vi "000_DataEmulator.vi"(11 "Queue Ref In":T1={"UI"=refnum, "Message"=refnum, "Data"=refnum, "Caller"=refnum, "Name"="000 Common", "Data Path"=path "", "Class Path"=path "", "SubPanel"=refnum, "Project Name"="", "MNT"="", "Title"="", "Data Source"=refnum, "Queue List"={}, "VI"=refnum, "UE"=refnum}) -> ()   [LabVIEW 2020]
doc: "000_DataEmulator.vi"
uses:
  Alin/QMH/000 Module Data Type.ctl
  Alin/QMH/Queue Message.ctl
  9999 SubVI/Global/Data Global/SDQ Data Type.ctl
  <vilib>/Utility/miscctls.llb/LVRowAndColumnUnsignedTypeDef.ctl
panel:
  in  "Delete":bool
  in  "Export":bool
  in  "Data Load":bool
  in  "Source Edit":bool
  out "Num":i32
  in  "Input":string
  in  "Panel Show":bool
  in  "Source List":i32[](listbox)
  in  "Delay(ms)":u32(slide)=250 min=5 max=2000 step=1 scale=5.0..2000.0
  in  "Simulation Start":bool
  in  "Data List":i32(listbox)
  out "Name":string
  out "Active ID":string
  out "Type":enum32{"decimal", "bool"}(tab)
  out "Unit":string
  in  "Type":enum16{"Sin"}(ring)
  in  "Single Simulation Start":bool
  in  "Value":sgl(slide)=250.0 min=0 max=1 scale=0.0..1.0 scale format="%#.6f"
  in  "Bool":bool
  out "Data":T2
  out "Count":u32
  out "Elapsed time(ms)":u32
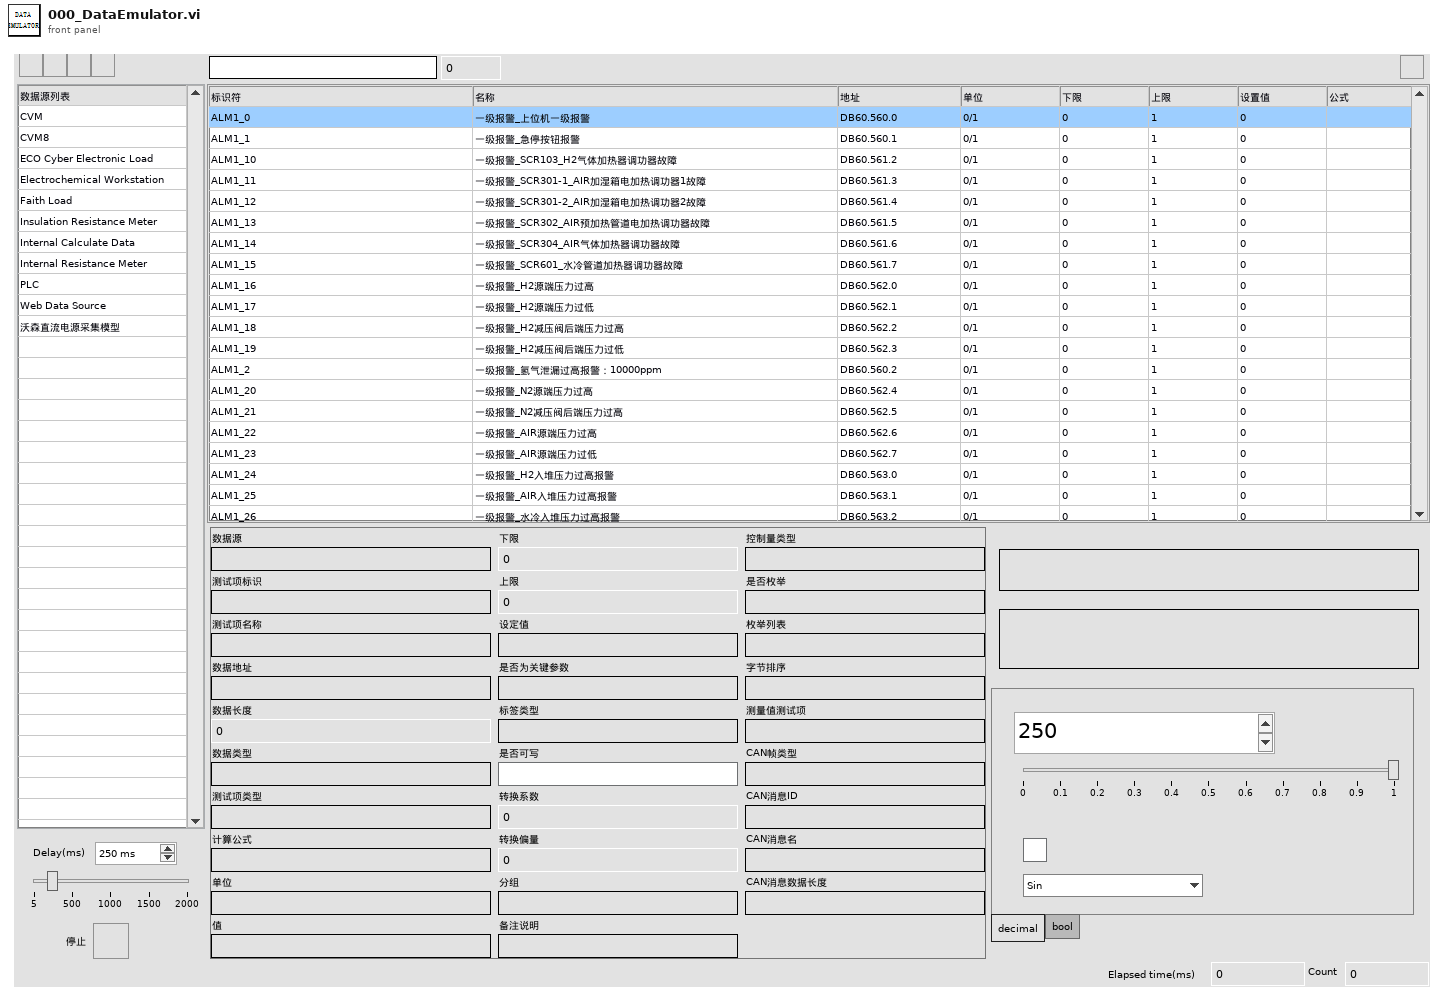
[diagram p1: front panel]
types:
  T1 = typedef "000 Module Data Type.ctl" = cluster{"UI":refnum<queue>, "Message":refnum<queue>, "Data":refnum<queue>, "Caller":refnum<queue>, "Name":string, "Data Path":path, "Class Path":path, "SubPanel":refnum<vi>, "Project Name":string, "MNT":string, "Title":string, "Data Source":refnum<queue>, "Queue List":map{string, refnum<queue>}, "VI":refnum<vi>, "UE":refnum<user-event>}
  T2 = typedef "SDQ Data Type.ctl" = cluster{"CAN Length":string, "CAN Name":string, "CAN ID":string, "CAN Type":string, "Test Item":string, "Byte Order":string, "Instruction":string, "Control Type":string, "Group":string, "Offset":dbl, "Coefficient":dbl, "Write Enable":bool, "Lable Type":string, "Key?":string, "Set Value":string, "Upper":dbl, "Lower":dbl, "Unit":string, "Formula":string, "Test Item Type":string, "Length":i32, "Address":string, "Name":string, "Identifier":string, "Data Type":string, "Enumerate?":string, "Enumerate List":string, "Data":string, "Source":string}
  T3 = typedef "LVRowAndColumnUnsignedTypeDef.ctl" = cluster{"Row":u32, "Column":u32}
  T4 = cluster{"Queue":T1, "Delay":cluster{"Count Time(ms)":u32, "Delay Time(ms)":u32, "Next":string}, "Data":map{string, T2}, "Start":bool, "Type":map{string, string}, "Source List":refnum<vi>, "TData":map{string, T2}, "Title":string[], "Source":map{string, string[]}, "Data List":refnum<vi>, "Value":refnum<vi>, "AID":string}
  T5 = cluster{"Name":string, "Type":map{string, string}}
  T6 = typedef "eventvkey.ctl" = enum16{"ASCII", "Enter", "Return", "Shift", "Ctrl", "Alt", "Cmd", "Opt", "Caps", "NumLock", "Clear", "Break", "Up", "Down", "Left", "Right", "Insert", "Delete", "Home", "End", "PageUp", "PageDown", "Escape", "Help", "Pause", "ScrollLock", "F1", "F2", "F3", "F4", "F5", "F6", "F7", "F8", "F9", "F10", "F11", "F12", "F13", "F14", "F15", "F16", "F17", "F18", "F19", "F20", "F21", "F22", "F23", "F24", "Play", "VolumeUp", "VolumeDown", "Mute", "Two Byte Char"}
  T7 = cluster{"Shift":bool, "Ctrl":bool, "Alt":bool, "Cmd":bool, "Opt":bool}
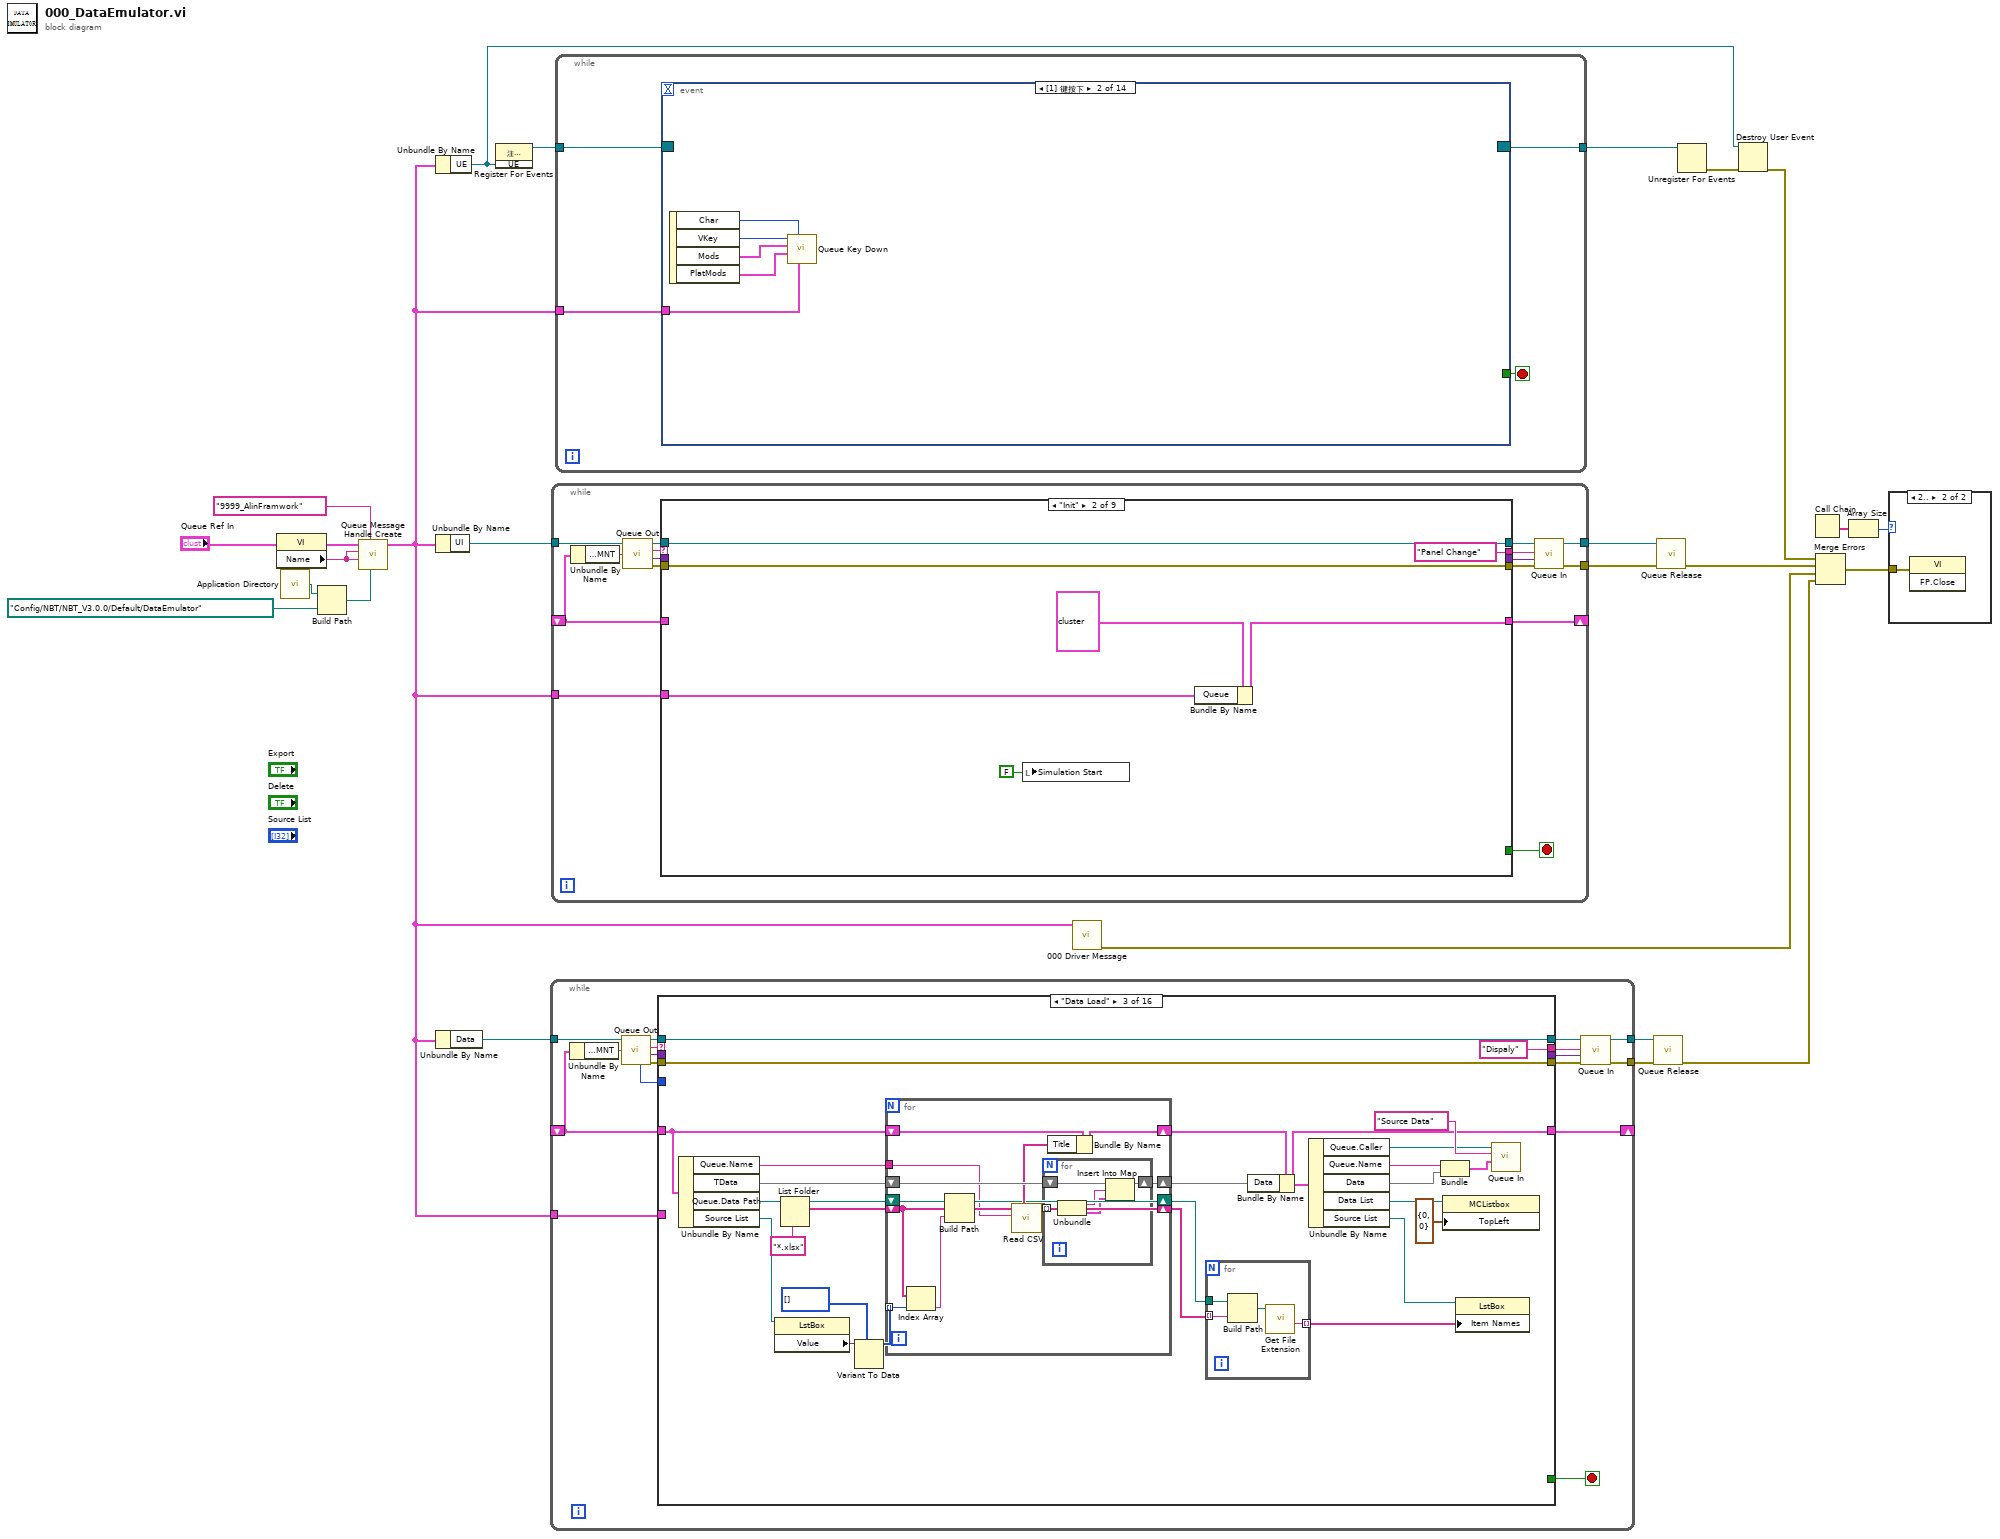
[diagram p0: block diagram]
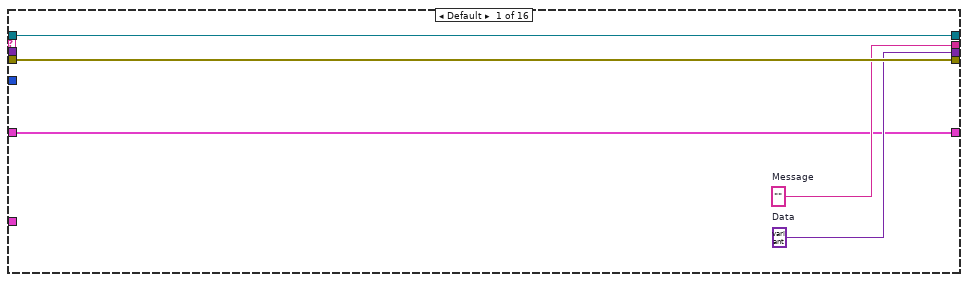
[diagram p2: hidden frame]
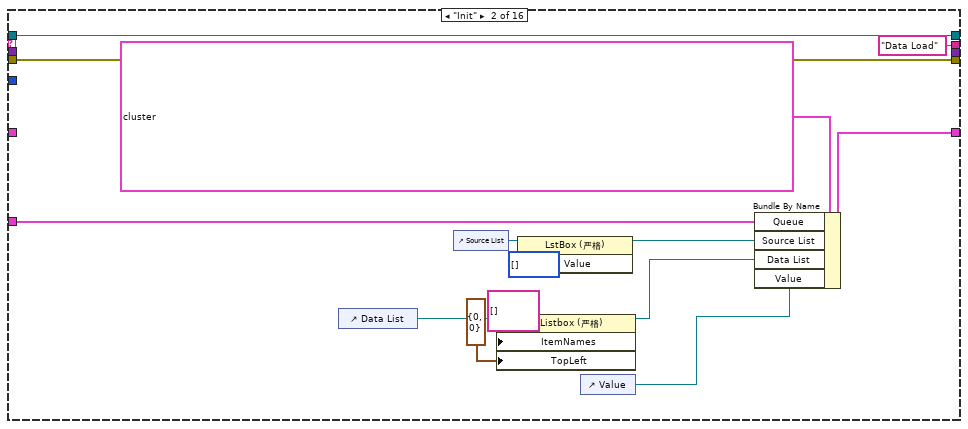
[diagram p3: hidden frame]
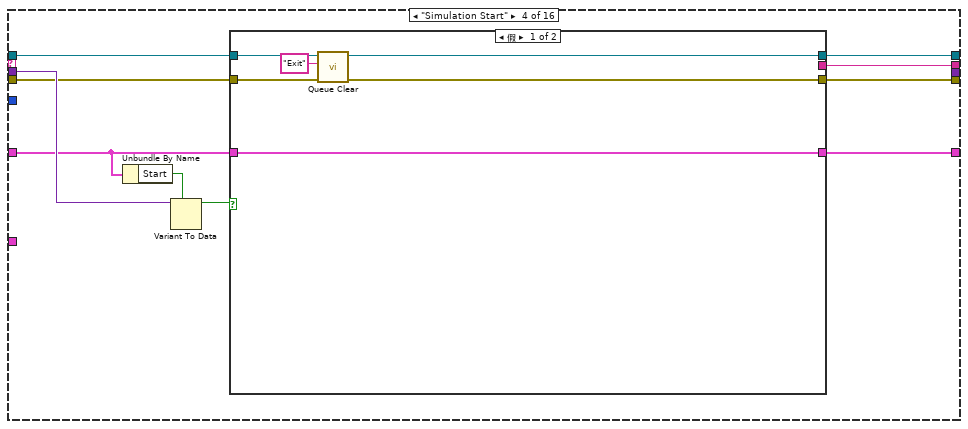
[diagram p4: hidden frame]
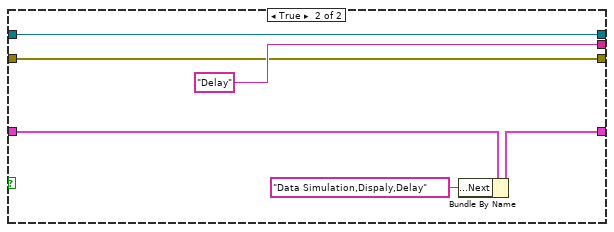
[diagram p5: hidden frame]
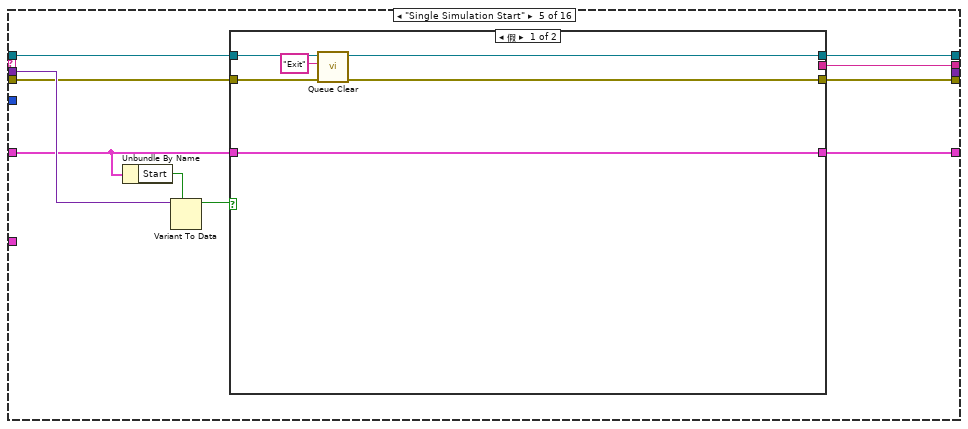
[diagram p6: hidden frame]
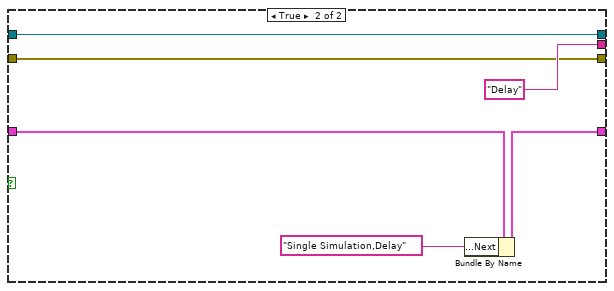
[diagram p7: hidden frame]
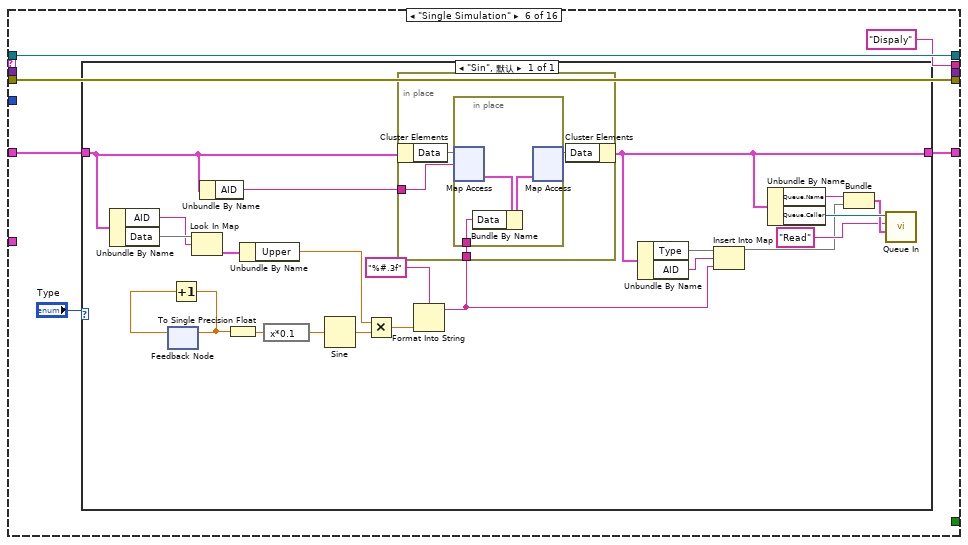
[diagram p8: hidden frame]
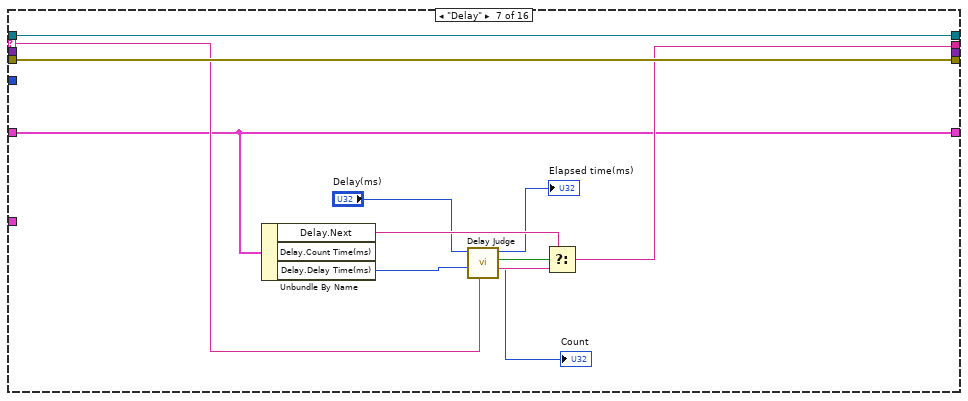
[diagram p9: hidden frame]
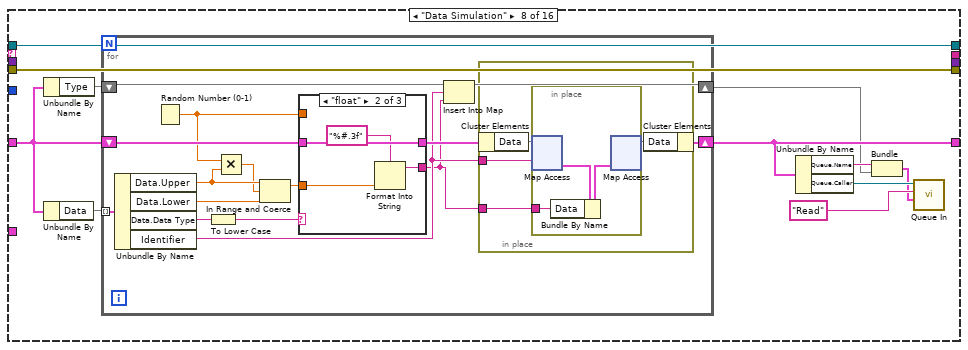
[diagram p10: hidden frame]
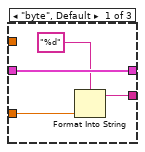
[diagram p11: hidden frame]
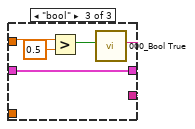
[diagram p12: hidden frame]
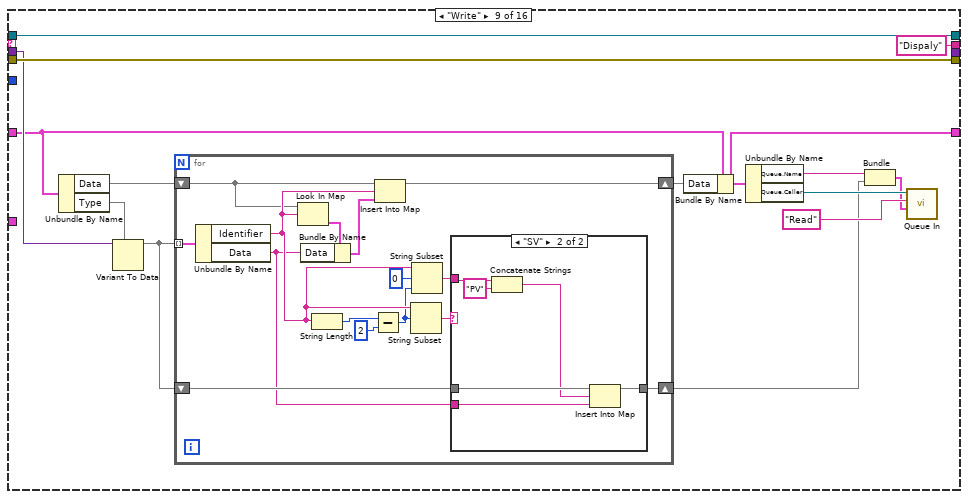
[diagram p13: hidden frame]
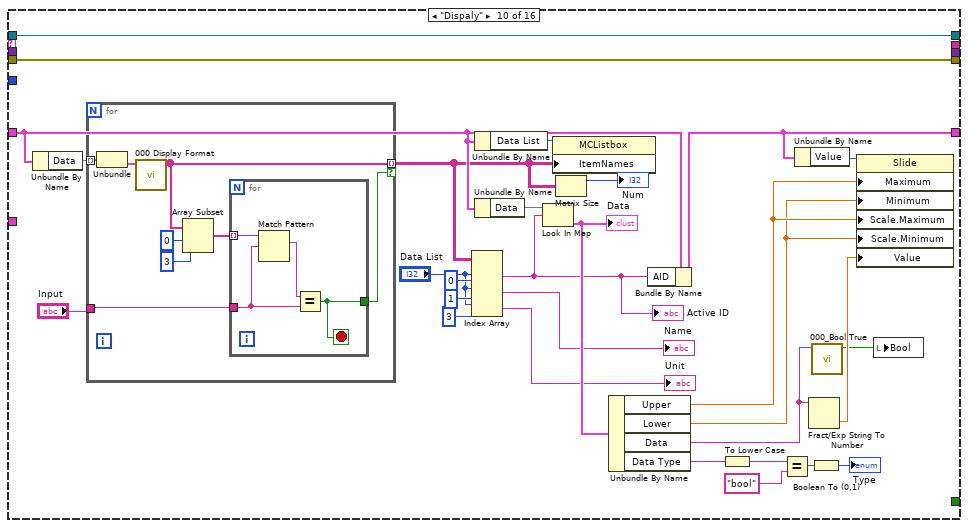
[diagram p15: hidden frame]
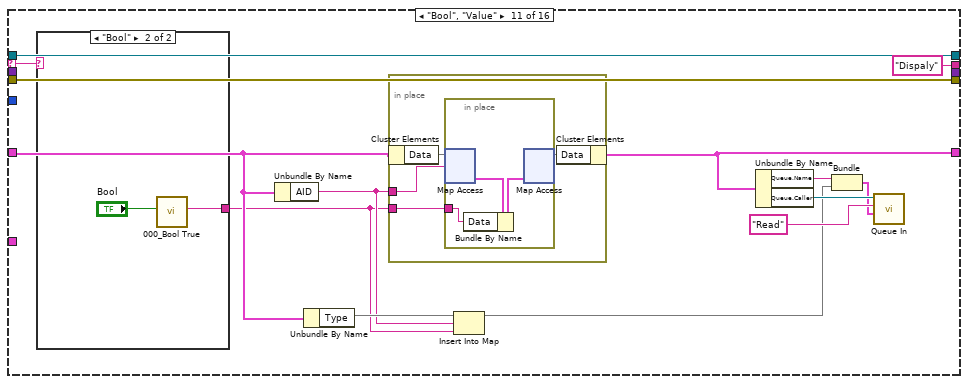
[diagram p16: hidden frame]
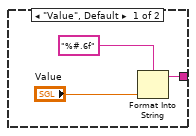
[diagram p17: hidden frame]
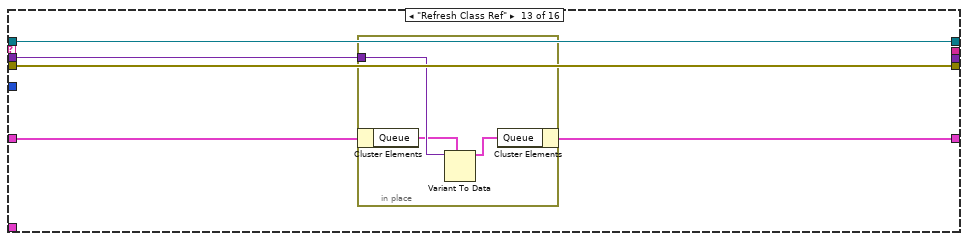
[diagram p19: hidden frame]
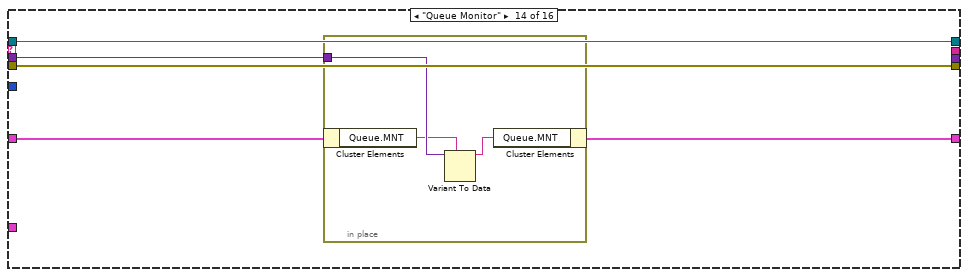
[diagram p20: hidden frame]
diagram:
  n1 = property class="VI"() -> ("Name"=w5:string)  [unwired: 2 in, 2 out]
  n2 = call <vilib>:"Application Directory.vi"() -> ("Application Directory"=w3:path)
  n3 = Build Path(base path=w3, name or relative path=path "Config/NBT/NBT_V3.0.0/Default/DataEmulator" ("名称或相对路径")) -> (appended path=w1:path)
  n4 = call "Queue Message Handle Create.vi"("Data Path"=w1, "Project Name"="9999_AlinFramwork", "Name"=w5, "Title"=w5, "Queue Ref In"="Queue Ref In") -> ("Queue Ref Out"=w6:T1)  [unwired: 5 in, 1 out]
  n5 = Unbundle By Name(w6) -> ("UE"=w8:refnum<user-event>)
  n6 = Unbundle By Name(w6) -> ("UI"=w19:refnum<queue>)
  n7 = Unbundle By Name(w6) -> ("Data"=w11:refnum<queue>)
  n8 = register-events(w8) -> (reference out=w24:refnum<event-registration>)  [unwired: 2 in, 1 out]
  n9 = while {
    tunnel: w11 -> [w37]
    tunnel: [w34] -> w13
    tunnel: [w33] -> w12
    shift-right: [w29] -> _
    shift-left: _ -> [w26]
    tunnel: w6 -> [w25]
    stop <- w41 stop-if-true
    n10 = Unbundle By Name(w26) -> ("Queue.MNT"=w27:string)
    n11 = call "Queue Out.vi"("Monitor"=w27, "Queue In"=w37) -> ("error out"=w40:errorcluster, "Data"=w38:variant, "Message"=w39:string, "Queue Out"=w36:refnum<queue>, "Queue NUmber"=w28:i32)  [unwired: 5 in]
    n12 = case shown="\"Data Load\"" w39 {
      selector: w39 -> [_ _ _ _ _ _ w193 _ _ _ w335 _ _ _ _ _]
      tunnel: w36 -> [w46 w60 w65 w116 w138 w159 w199 w210 w260 w311 w337 w352 w357 w365 w373 w377]
      tunnel: w40 -> [w45 w59 w88 w114 w136 w158 w198 w209 w259 w310 w336 w351 w356 w364 w371 w378]
      tunnel: [w46 w60 w65 w115 w137 w159 w199 w210 w260 w311 w337 w352 w357 w365 w372 w377] -> w35
      tunnel: [w45 w59 w88 w113 w135 w158 w198 w209 w259 w310 w336 w351 w356 w364 w370 w378] -> w32
      tunnel: [w44 "Data Load" ("Next") "Dispaly" ("Next") w117 w139 "Dispaly" ("Next") w194 _ "Dispaly" ("Next") _ "Dispaly" ("Next") _ _ _ "Quit" _] -> w31
      tunnel: [_ _ _ _ _ _ _ _ _ _ _ _ _ _ _ TRUE] -> w41
      tunnel: [w43 _ _ _ _ _ _ _ _ _ _ _ _ _ _ _] -> w30
      tunnel: w38 -> [_ _ _ w119 w141 _ _ _ w258 _ _ _ w353 w361 _ _]
      tunnel: [w42 w56 w73 w110 w132 w155 w192 w205 w248 w296 w330 w350 w354 w362 w369 w375] -> w29
      tunnel: w26 -> [w42 _ w67 w111 w133 w156 w192 w207 w255 w298 w329 w350 w355 w363 w369 w375]
      tunnel: w28 -> [_ _ _ _ _ _ _ _ _ _ _ _ _ _ _ _]
      tunnel: w25 -> [_ w55 _ _ _ _ _ _ _ _ _ _ _ _ _ _]
      frame Default {
        w43 = variant  # Data
        w44 = ""  # Message
      }
      frame "Init" {
        n13 = control-ref of="Data List"() -> (w51:refnum<vi>)
        n14 = control-ref of="Source List"() -> (w54:refnum<vi>)
        n15 = property class="MCListbox (严格)"(reference=w51, "ItemNames"=string[][] [] ("项名"), "TopLeft"=T3 {"Row"=0, "Column"=0} ("左上可见单元格")) -> (reference out=w50:refnum<vi>)  [unwired: 1 in, 1 out]
        n16 = property class="LstBox (严格)"(reference=w54, "Value"=i32[] [] ("值")) -> (reference out=w53:refnum<vi>)  [unwired: 1 in, 1 out]
        n17 = control-ref of="Value"() -> (w47:refnum<vi>)
        n18 = Bundle By Name(cluster=T4 {"Queue"={"UI"=refnum, "Message"=refnum, "Data"=refnum, "Caller"=refnum, "Name"="000 Common", "Data Path"=path "", "Class Path"=path "", "SubPanel"=refnum, "Project Name"="", "MNT"="", "Title"="", "Data Source"=refnum, "Queue List"={}, "VI"=refnum, "UE"=refnum}, "Delay"={"Count Time(ms)"=250, "Delay Time(ms)"=50, "Next"="Data Simulation,Dispaly,Delay"}, "Data"={}, "Start"=FALSE, "Type"={}, "Source List"=refnum, "TData"={}, "Title"=[], "Source"={}, "Data List"=refnum, "Value"=refnum, "AID"=""}, "Queue"=w55, "Source List"=w53, "Data List"=w50, "Value"=w47) -> (w56:T4)
      }
      frame "Data Load" {
        n19 = Unbundle By Name(w67) -> ("Queue.Name"=w72:string, "TData"=w85:map{string, T2}, "Queue.Data Path"=w87:path, "Source List"=w83:refnum<vi>)
        n20 = property class="LstBox"(reference=w83) -> ("Value"=w82:variant)  [unwired: 1 in, 2 out]
        n21 = List Folder(path=w87, pattern="*.xlsx" ("类型")) -> (path out=w86:path, filenames=w79:string[])  [unwired: 2 in, 2 out]
        n22 = Variant To Data(type=i32[] [] ("Source List"), Variant=w82) -> (data=w80:i32[])  [unwired: 1 in, 1 out]
        n23 = for {
          shift-right: [w102] -> w84
          shift-left: w85 -> [w103]
          tunnel: w80 -> [w101] mode=indexing
          tunnel: w72 -> [w93]
          shift-right: [w100] -> w70
          shift-left: w79 -> [w100]
          shift-right: [w95] -> w71
          shift-left: w86 -> [w95]
          shift-right: [w98] -> w66
          shift-left: w67 -> [w99]
          n24 = Index Array(array=w100, index=w101) -> (element=w96:string)
          n25 = Build Path(base path=w95, name or relative path=w96) -> (appended path=w94:path)
          n26 = call "Read CSV.vi"("Source"=w93, "Data Path"=w94) -> ("Identifiers Out"=w104:map{string, T2}, "Title"=w97:string[])  [unwired: 2 in, 6 out]
          n27 = for {
            tunnel: w104 -> [w107] mode=indexing
            shift-right: [w108] -> w102
            shift-left: w103 -> [w109]
            n28 = Unbundle(w107) -> ("Identifier"=w105:string, "Data"=w106:T2)
            n29 = Insert Into Map(map in=w109, key=w105, value=w106) -> (map out=w108:map{string, T2})  [unwired: 2 out]
          }
          n30 = Bundle By Name(cluster=w99, "Title"=w97) -> (w98:T4)
        }
        n31 = for {
          tunnel: w71 -> [w92]
          tunnel: w70 -> [w91] mode=indexing
          tunnel: [w89] -> w69 mode=indexing
          n32 = Build Path(base path=w92, name or relative path=w91) -> (appended path=w90:path)
          n33 = call <vilib>:"Get File Extension.vi"("file"=w90) -> ("filename without extension"=w89:string)  [unwired: 6 in, 4 out]
        }
        n34 = Bundle By Name(cluster=w66, "Data"=w84) -> (w73:T4)
        n35 = Unbundle By Name(w73) -> ("Queue.Caller"=w74:refnum<queue>, "Queue.Name"=w78:string, "Data"=w76:map{string, T2}, "Data List"=w62:refnum<vi>, "Source List"=w63:refnum<vi>)
        n36 = Bundle("Name"=w78, "Data"=w76) -> (w77:cluster{"Name":string, "Data":map{string, T2}})  [unwired: 1 in]
        n37 = property class="MCListbox"(reference=w62, "TopLeft"=T3 {"Row"=0, "Column"=0} ("左上可见单元格")) -> ()  [unwired: 1 in, 2 out]
        n38 = property class="LstBox"(reference=w63, "Item Names"=w69) -> ()  [unwired: 1 in, 2 out]
        n39 = call "Queue In.vi"("Data"=w77, "Message"="Source Data", "Queue In"=w74) -> ()  [unwired: 7 in, 2 out]
      }
      frame "Simulation Start" {
        n40 = Unbundle By Name(w111) -> ("Start"=w112:bool)
        n41 = Variant To Data(type=w112, Variant=w119) -> (data=w118:bool)  [unwired: 1 in, 1 out]
        n42 = case shown="假" w118 {
          tunnel: [_ "Delay" ("Next")] -> w117
          tunnel: w116 -> [w123 w130]
          tunnel: [w122 w130] -> w115
          tunnel: w114 -> [w125 w129]
          tunnel: [w124 w129] -> w113
          tunnel: w111 -> [w120 w128]
          tunnel: [w120 w127] -> w110
          frame False {
            n43 = call "Queue Clear.vi"("error in (no error)"=w125, "Filter"="Exit", "Queue In"=w123) -> ("error out"=w124:errorcluster, "Queue Out"=w122:refnum<queue>)  [unwired: 7 in]
          }
          frame True {
            n44 = Bundle By Name(cluster=w128, "Delay.Next"="Data Simulation,Dispaly,Delay") -> (w127:T4)
          }
        }
      }
      frame "Single Simulation Start" {
        n45 = Unbundle By Name(w133) -> ("Start"=w134:bool)
        n46 = Variant To Data(type=w134, Variant=w141) -> (data=w140:bool)  [unwired: 1 in, 1 out]
        n47 = case shown="假" w140 {
          tunnel: [_ "Delay" ("Next")] -> w139
          tunnel: w138 -> [w145 w152]
          tunnel: [w144 w152] -> w137
          tunnel: w136 -> [w147 w151]
          tunnel: [w146 w151] -> w135
          tunnel: w133 -> [w142 w150]
          tunnel: [w142 w149] -> w132
          frame False {
            n48 = call "Queue Clear.vi"("error in (no error)"=w147, "Filter"="Exit", "Queue In"=w145) -> ("error out"=w146:errorcluster, "Queue Out"=w144:refnum<queue>)  [unwired: 7 in]
          }
          frame True {
            n49 = Bundle By Name(cluster=w150, "Delay.Next"="Single Simulation,Delay") -> (w149:T4)
          }
        }
      }
      frame "Single Simulation" {
        n50 = case shown="\"Sin\", 默认" "Type" {
          tunnel: w156 -> [w169]
          tunnel: [w161] -> w155
          frame "Sin", Default {
            n51 = Unbundle By Name(w169) -> ("AID"=w171:string, "Data"=w177:map{string, T2})
            n52 = feedback #1() -> (w180:dbl)  [unwired: 1 in]
            n53 = Increment(x=w180) -> (x+1=w179:dbl)
            n54 = feedback-in #1(w179) -> ()
            n55 = Look In Map(map=w177, key=w171) -> (value=w176:T2)  [unwired: 1 in, 1 out]
            n56 = Unbundle By Name(w169) -> ("AID"=w168:string)
            n57 = To Single Precision Float(number=w179) -> (single precision float=w181:sgl)
            n58 = Unbundle By Name(w176) -> ("Upper"=w175:dbl)
            n59 = expression code="x*0.1"(w181) -> (w172:sgl)
            n60 = Sine(x=w172) -> (sin(x)=w178:sgl)
            n61 = Multiply(x=w175, y=w178) -> (x*y=w173:dbl)
            n62 = Format Into String(format string="%#.3f" ("格式字符串"), w173) -> (resulting string=w166:string)  [unwired: 2 in, 1 out]
            n63 = in-place {
              in-place-border: w166 -> [w183]
              in-place-border: w168 -> [w182]
              n64 = in-place-cluster #2(w169) -> ("Data"=w185:map{string, T2})
              n65 = in-place {
                in-place-border: w183 -> [w186]
                n66 = in-place-map #3(w185, w182) -> (w188:T2)  [unwired: 1 in, 1 out]
                n67 = Bundle By Name(cluster=w188, "Data"=w186) -> (w187:T2)
                n68 = in-place-map #3(w187) -> (w184:map{string, T2})  [unwired: 1 in, 2 out]
              }
              n69 = in-place-cluster #2("Data"=w184) -> (w161:T4)
            }
            n70 = Unbundle By Name(w161) -> ("Type"=w170:map{string, string}, "AID"=w167:string)
            n71 = Insert Into Map(map in=w170, key=w167, value=w166) -> (map out=w160:map{string, string})  [unwired: 2 out]
            n72 = Unbundle By Name(w161) -> ("Queue.Name"=w164:string, "Queue.Caller"=w165:refnum<queue>)
            n73 = Bundle("Name"=w164, "Type"=w160) -> (w163:T5)  [unwired: 1 in]
            n74 = call "Queue In.vi"("Data"=w163, "Message"="Read", "Queue In"=w165) -> ()  [unwired: 7 in, 2 out]
          }
        }
      }
      frame "Delay" {
        n75 = Unbundle By Name(w192) -> ("Delay.Next"=w197:string, "Delay.Delay Time(ms)"=w195:u32)  [unwired: 1 out]
        n76 = call "Delay Judge.vi"("Delay Time(ms)"=w195, "Count Time(ms)"="Delay(ms)") -> ("Count"=→"Count":u32, "Time Out?"=w196:bool, "Elapsed time(ms)"=→"Elapsed time(ms)":u32)  [unwired: 5 in, 2 out]
        n77 = Select(t=w197, s=w196, f=w193) -> (s? t:f=w194:string)
      }
      frame "Data Simulation" {
        n78 = Unbundle By Name(w207) -> ("Type"=w206:map{string, string})
        n79 = Unbundle By Name(w207) -> ("Data"=w208:map{string, T2})
        n80 = for {
          tunnel: w208 -> [w224] mode=indexing
          shift-right: [w213] -> w205
          shift-left: w207 -> [w222]
          shift-right: [w215] -> w200
          shift-left: w206 -> [w214]
          n81 = Unbundle By Name(w224) -> ("Data.Upper"=w218:dbl, "Data.Lower"=w220:dbl, "Data.Data Type"=w221:string, "Identifier"=w212:string)
          n82 = Random Number (0-1)() -> (number: 0 to 1=w216:dbl)
          n83 = To Lower Case(string=w221) -> (all lower case string=w225:string)
          n84 = Multiply(x=w216, y=w218) -> (x*y=w217:dbl)
          n85 = In Range and Coerce(upper limit=w218, x=w217, lower limit=w220) -> (coerced(x)=w219:dbl)  [unwired: 1 out]
          n86 = case shown="\"float\"" w225 {
            tunnel: w222 -> [w236 w240 w245]
            tunnel: [w236 w240 w245] -> w223
            tunnel: w219 -> [w234 w238 _]
            tunnel: [w233 w237 w241] -> w211
            tunnel: w216 -> [_ _ w244]
            frame "byte", Default {
              n87 = Format Into String(format string="%d" ("格式字符串"), w234) -> (resulting string=w233:string)  [unwired: 2 in, 1 out]
            }
            frame "float" {
              n88 = Format Into String(format string="%#.3f" ("格式字符串"), w238) -> (resulting string=w237:string)  [unwired: 2 in, 1 out]
            }
            frame "bool" {
              n89 = Greater?(x=w244, y=0.5) -> (0:w242:bool)
              n90 = call "000_Bool True.vi"("Value"=w242) -> ("String Out"=w241:string)  [unwired: 8 in, 2 out]
            }
          }
          n91 = Insert Into Map(map in=w214, key=w212, value=w211) -> (map out=w215:map{string, string})  [unwired: 2 out]
          n92 = in-place {
            in-place-border: w212 -> [w227]
            in-place-border: w211 -> [w226]
            n93 = in-place-cluster #4(w223) -> ("Data"=w229:map{string, T2})
            n94 = in-place {
              in-place-border: w226 -> [w230]
              n95 = in-place-map #5(w229, w227) -> (w232:T2)  [unwired: 1 in, 1 out]
              n96 = Bundle By Name(cluster=w232, "Data"=w230) -> (w231:T2)
              n97 = in-place-map #5(w231) -> (w228:map{string, T2})  [unwired: 1 in, 2 out]
            }
            n98 = in-place-cluster #4("Data"=w228) -> (w213:T4)
          }
        }
        n99 = Unbundle By Name(w205) -> ("Queue.Name"=w202:string, "Queue.Caller"=w204:refnum<queue>)
        n100 = Bundle("Name"=w202, "Type"=w200) -> (w201:T5)  [unwired: 1 in]
        n101 = call "Queue In.vi"("Data"=w201, "Message"="Read", "Queue In"=w204) -> ()  [unwired: 7 in, 2 out]
      }
      frame "Write" {
        n102 = Unbundle By Name(w255) -> ("Data"=w257:map{string, T2}, "Type"=w256:map{string, string})
        n103 = Variant To Data(type=w256, Variant=w258) -> (data=w247:map{string, string})  [unwired: 1 in, 1 out]
        n104 = for {
          tunnel: w247 -> [w275] mode=indexing
          shift-right: [w270] -> w254
          shift-left: w257 -> [w264]
          shift-right: [w262] -> w246
          shift-left: w247 -> [w263]
          n105 = Unbundle By Name(w275) -> ("Identifier"=w269:string, "Data"=w261:string)
          n106 = Look In Map(map=w264, key=w269) -> (value=w274:T2)  [unwired: 1 in, 1 out]
          n107 = Bundle By Name(cluster=w274, "Data"=w261) -> (w273:T2)
          n108 = String Length(string=w269) -> (length=w272:i32)
          n109 = Subtract(x=w272, y=2 ("偏移量(0)")) -> (x-y=w266:i32)
          n110 = Insert Into Map(map in=w264, key=w269, value=w273) -> (map out=w270:map{string, T2})  [unwired: 2 out]
          n111 = String Subset(string=w269, offset (0)=w266) -> (substring=w268:string)  [unwired: 1 in]
          n112 = String Subset(string=w269, offset (0)=0 ("偏移量(0)"), length (rest)=w266) -> (substring=w267:string)
          n113 = case shown="\"SV\"" w268 {
            tunnel: w267 -> [_ w282]
            tunnel: w263 -> [w276 w280]
            tunnel: [w276 w279] -> w262
            tunnel: w261 -> [_ w277]
            frame Default {
            }
            frame "SV" {
              n114 = Concatenate Strings(w282, "PV" ("字符串")) -> (w278:string)
              n115 = Insert Into Map(map in=w280, key=w278, value=w277) -> (map out=w279:map{string, string})  [unwired: 2 out]
            }
          }
        }
        n116 = Bundle By Name(cluster=w255, "Data"=w254) -> (w248:T4)
        n117 = Unbundle By Name(w248) -> ("Queue.Name"=w250:string, "Queue.Caller"=w252:refnum<queue>)
        n118 = Bundle("Name"=w250, "Type"=w246) -> (w249:T5)  [unwired: 1 in]
        n119 = call "Queue In.vi"("Data"=w249, "Message"="Read", "Queue In"=w252) -> ()  [unwired: 7 in, 2 out]
      }
      frame "Dispaly" {
        n120 = Unbundle By Name(w298) -> ("Data"=w309:map{string, T2})
        n121 = for {
          tunnel: [w314] -> w292 mode=indexing if=w315
          tunnel: "Input" -> [w316]
          tunnel: w309 -> [w313] mode=indexing
          n122 = Unbundle(w313) -> ("Data"=w312:T2)  [unwired: 1 out]
          n123 = call "000 Display Format.vi"("Data"=w312) -> ("Data"=w314:string[])  [unwired: 10 in]
          n124 = Array Subset(array=w314, index=0 ("索引"), length=3 ("长度")) -> (w317:string[])
          n125 = for {
            tunnel: w317 -> [w323] mode=indexing
            tunnel: w316 -> [w321]
            tunnel: [w320] -> w315
            stop <- w320 stop-if-true
            n126 = Match Pattern(string=w323, regular expression=w321) -> (match substring=w322:string)  [unwired: 1 in, 3 out]
            n127 = Equal?(x=w322, y=w321) -> (x = y?=w320:bool)
          }
        }
        n128 = Index Array(array=w292, index (row) #1="Data List", index (col) #1=0 ("禁用的索引 (列)"), index (row) #2="Data List", index (col) #2=1 ("禁用的索引 (列)"), index (row) #3="Data List", index (col) #3=3 ("禁用的索引 (列)")) -> (element #1=w290:string, element #2=→"Name":string, element #3=→"Unit":string)
        "Active ID" <- w290
        n129 = Unbundle By Name(w298) -> ("Data List"=w307:refnum<vi>)
        n130 = Unbundle By Name(w298) -> ("Data"=w306:map{string, T2})
        n131 = Look In Map(map=w306, key=w290) -> (value=w304:T2)  [unwired: 1 in, 1 out]
        "Data" <- w304
        n132 = property class="MCListbox"(reference=w307, "ItemNames"=w292) -> ()  [unwired: 1 in, 2 out]
        n133 = Matrix Size(0:w292) -> (1:→"Num":i32)  [unwired: 1 out]
        n134 = Unbundle By Name(w304) -> ("Upper"=w294:dbl, "Lower"=w293:dbl, "Data"=w284:string, "Data Type"=w303:string)
        n135 = Bundle By Name(cluster=w298, "AID"=w290) -> (w296:T4)
        n136 = To Lower Case(string=w303) -> (all lower case string=w301:string)
        n137 = Equal?(x=w301, y="bool") -> (x = y?=w300:bool)
        n138 = Unbundle By Name(w296) -> ("Value"=w297:refnum<vi>)
        n139 = Fract/Exp String To Number(string=w284) -> (number=w295:dbl)  [unwired: 3 in, 1 out]
        n140 = Boolean To (0,1)(Boolean=w300) -> (0, 1=→"Type":i16)
        n141 = call "000_Bool True.vi"("Bool String"=w284) -> ("True"=w283:bool)  [unwired: 8 in, 2 out]
        n142 = property class="Slide"(reference=w297, "Maximum"=w294, "Minimum"=w293, "Scale.Maximum"=w294, "Scale.Minimum"=w293, "Value"=w295) -> ()  [unwired: 1 in, 2 out]
        n143 = local write "Bool"(w283) -> ()
      }
      frame "Bool", "Value" {
        n144 = case shown="\"Bool\"" w335 {
          tunnel: [w345 w348] -> w325
          frame "Value", Default {
            n145 = Format Into String(format string="%#.6f" ("格式字符串"), "Value") -> (resulting string=w345:string)  [unwired: 2 in, 1 out]
          }
          frame "Bool" {
            n146 = call "000_Bool True.vi"("Value"="Bool") -> ("String Out"=w348:string)  [unwired: 8 in, 2 out]
          }
        }
        n147 = Unbundle By Name(w329) -> ("AID"=w326:string)
        n148 = Unbundle By Name(w329) -> ("Type"=w328:map{string, string})
        n149 = in-place {
          in-place-border: w326 -> [w339]
          in-place-border: w325 -> [w338]
          n150 = in-place-cluster #6(w329) -> ("Data"=w341:map{string, T2})
          n151 = in-place {
            in-place-border: w338 -> [w342]
            n152 = in-place-map #7(w341, w339) -> (w344:T2)  [unwired: 1 in, 1 out]
            n153 = Bundle By Name(cluster=w344, "Data"=w342) -> (w343:T2)
            n154 = in-place-map #7(w343) -> (w340:map{string, T2})  [unwired: 1 in, 2 out]
          }
          n155 = in-place-cluster #6("Data"=w340) -> (w330:T4)
        }
        n156 = Insert Into Map(map in=w328, key=w326, value=w325) -> (map out=w327:map{string, string})  [unwired: 2 out]
        n157 = Unbundle By Name(w330) -> ("Queue.Name"=w332:string, "Queue.Caller"=w334:refnum<queue>)
        n158 = Bundle("Name"=w332, "Type"=w327) -> (w331:T5)  [unwired: 1 in]
        n159 = call "Queue In.vi"("Data"=w331, "Message"="Read", "Queue In"=w334) -> ()  [unwired: 7 in, 2 out]
      }
      frame "====System====" {
      }
      frame "Refresh Class Ref" {
        n160 = in-place {
          in-place-border: w353 -> [w360]
          n161 = in-place-cluster #8(w355) -> ("Queue"=w359:T1)
          n162 = Variant To Data(type=w359, Variant=w360) -> (data=w358:T1)  [unwired: 1 in, 1 out]
          n163 = in-place-cluster #8("Queue"=w358) -> (w354:T4)
        }
      }
      frame "Queue Monitor" {
        n164 = in-place {
          in-place-border: w361 -> [w368]
          n165 = in-place-cluster #9(w363) -> ("Queue.MNT"=w367:string)
          n166 = Variant To Data(type=w367, Variant=w368) -> (data=w366:string)  [unwired: 1 in, 1 out]
          n167 = in-place-cluster #9("Queue.MNT"=w366) -> (w362:T4)
        }
      }
      frame "Exit" {
        n168 = call "Queue Clear.vi"("error in (no error)"=w371, "Queue In"=w373) -> ("error out"=w370:errorcluster, "Queue Out"=w372:refnum<queue>)  [unwired: 8 in]
      }
      frame "Quit" {
      }
    }
    n169 = call "Queue In.vi"("error in (no error)"=w32, "Data"=w30, "Message"=w31, "Queue In"=w35) -> ("error out"=w33:errorcluster, "Queue Out"=w34:refnum<queue>)  [unwired: 6 in]
  }
  n170 = while {
    tunnel: w19 -> [w390]
    tunnel: [w387] -> w21
    tunnel: [w386] -> w20
    shift-right: [w382] -> _
    shift-left: _ -> [w381]
    tunnel: w6 -> [w379]
    stop <- w394 stop-if-true
    n171 = Unbundle By Name(w381) -> ("Queue.MNT"=w380:string)
    n172 = call "Queue Out.vi"("Monitor"=w380, "Queue In"=w390) -> ("error out"=w393:errorcluster, "Data"=w391:variant, "Message"=w392:string, "Queue Out"=w389:refnum<queue>)  [unwired: 5 in, 1 out]
    n173 = case shown="\"Init\"" w392 {
      selector: w392 -> [_ _ _ _ _ _ _ w440 _]
      tunnel: w389 -> [w399 w406 w409 w416 w421 w426 w434 w447 w453]
      tunnel: w393 -> [w398 w405 w408 w415 w420 w425 w433 w445 w454]
      tunnel: [w399 w406 w409 w416 w421 w426 w434 w446 w453] -> w388
      tunnel: [w398 w405 w408 w415 w420 w425 w433 w444 w454] -> w385
      tunnel: [w397 "Panel Change" ("Message") _ _ _ _ _ "Quit" _] -> w384
      tunnel: [_ _ _ _ _ _ _ _ TRUE] -> w394
      tunnel: [w396 _ _ _ _ _ _ _ _] -> w383
      tunnel: w391 -> [_ _ _ _ _ w422 w430 _ _]
      tunnel: [w395 w403 w407 w414 w419 w423 w431 w439 w451] -> w382
      tunnel: w381 -> [w395 _ w407 w414 w419 w424 w432 w439 w451]
      tunnel: w379 -> [_ w402 _ _ _ _ _ _ _]
      frame Default {
        w396 = variant  # Data
        w397 = ""  # Message
      }
      frame "Init" {
        n174 = local write "Simulation Start"(FALSE ("Simulation Start")) -> ()
        n175 = Bundle By Name(cluster=cluster{"Queue":T1} {"Queue"={"UI"=refnum, "Message"=refnum, "Data"=refnum, "Caller"=refnum, "Name"="000 Common", "Data Path"=path "", "Class Path"=path "", "SubPanel"=refnum, "Project Name"="", "MNT"="", "Title"="", "Data Source"=refnum, "Queue List"={}, "VI"=refnum, "UE"=refnum}}, "Queue"=w402) -> (w403:cluster{"Queue":T1})
      }
      frame "Panel Change" {
        n176 = call "MCList Adjust.vi"() -> ()  [unwired: 11 in, 1 out]
      }
      frame "Source Edit" {
        n177 = Unbundle By Name(w414) -> ("Queue.Data Path"=w413:path)
        n178 = call <vilib>:"Check if File or Folder Exists.vi"("path"=w413) -> ("error out"=w410:errorcluster, "file or folder exists?"=w412:bool, "dup path"=w411:path)  [unwired: 8 in]
        n179 = case shown="真" w412 {
          tunnel: w411 -> [_ w418]
          tunnel: w410 -> [_ w417]
          frame False {
          }
          frame True {
            n180 = call <vilib>:"Show in File System.vi"("error in (no error)"=w417, "file or directory path"=w418) -> ()  [unwired: 9 in, 1 out]
          }
        }
      }
      frame "====System====" {
      }
      frame "Refresh Class Ref" {
        n181 = in-place {
          in-place-border: w422 -> [w429]
          n182 = in-place-cluster #10(w424) -> ("Queue"=w428:T1)
          n183 = Variant To Data(type=w428, Variant=w429) -> (data=w427:T1)  [unwired: 1 in, 1 out]
          n184 = in-place-cluster #10("Queue"=w427) -> (w423:cluster{"Queue":T1})
        }
      }
      frame "Queue Monitor" {
        n185 = in-place {
          in-place-border: w430 -> [w437]
          n186 = in-place-cluster #11(w432) -> ("Queue.MNT"=w436:string)
          n187 = Variant To Data(type=w436, Variant=w437) -> (data=w435:string)  [unwired: 1 in, 1 out]
          n188 = in-place-cluster #11("Queue.MNT"=w435) -> (w431:cluster{"Queue":T1})
        }
      }
      frame "Exit" {
        n189 = Unbundle By Name(w439) -> ("Queue.Message"=w443:refnum<queue>, "Queue.Data"=w442:refnum<queue>, "Queue.UE"=w438:refnum<user-event>)
        n190 = Build Array(w443, w442) -> (w441:refnum<queue>[])
        n191 = Generate User Event(user event=w438, event data cluster=w440) -> ()  [unwired: 2 in, 2 out]
        n192 = for {
          tunnel: w441 -> [w450] mode=indexing
          tunnel: w440 -> [w449]
          n193 = call "Queue In.vi"("Message"=w449, "Queue In"=w450) -> ()  [unwired: 8 in, 2 out]
        }
        n194 = call "Queue Clear.vi"("error in (no error)"=w445, "Queue In"=w447) -> ("error out"=w444:errorcluster, "Queue Out"=w446:refnum<queue>)  [unwired: 8 in]
      }
      frame "Quit" {
      }
    }
    n195 = call "Queue In.vi"("error in (no error)"=w385, "Data"=w383, "Message"=w384, "Queue In"=w388) -> ("error out"=w386:errorcluster, "Queue Out"=w387:refnum<queue>)  [unwired: 6 in]
  }
  n196 = while {
    tunnel: w24 -> [w458]
    tunnel: [w456] -> w23
    tunnel: w6 -> [w455]
    stop <- w457 stop-if-true
    n197 = event shown="[1] 键按下" {
      selector: w458 -> [_ _ _ _ _ _ _ _ _ _ _ _ _ _]
      dyn-events: [_ _ _ _ _ _ _ _ _ _ _ _ _ _] -> w456
      timeout: _ -> [_ _ _ _ _ _ _ _ _ _ _ _ _ _]
      tunnel: [_ _ _ w467 _ _ _ _ _ _ _ _ _ _] -> w457
      tunnel: w455 -> [_ w462 w466 _ w472 w486 w489 w494 w498 w502 w505 w508 w513 w516]
      event Timeout {
        n198 = event-data() -> ()  [unwired: 1 in, 1 out]
      }
      event Key Down {
        n199 = event-data() -> ("Char"=w463:i16, "VKey"=w461:T6, "Mods"=w460:cluster{"Num Pad":bool, "Menu Key":bool}, "PlatMods"=w459:T7)  [unwired: 1 in]
        n200 = call "Queue Key Down.vi"("Queue Ref Out"=w462, "C"=w463, "Platform Key"=w459, "Group Key"=w460, "V Key"=w461) -> ()  [unwired: 6 in, 1 out]
      }
      event Panel Resize {
        n201 = event-data() -> ()  [unwired: 1 in, 1 out]
        n202 = Unbundle By Name(w466) -> ("Message"=w465:refnum<queue>)
        n203 = call "Queue In.vi"("Message"="Panel Change", "Queue In"=w465) -> ()  [unwired: 8 in, 2 out]
      }
      event User Event {
        n204 = event-data() -> ("Message"=w469:string)  [unwired: 1 in]
        n205 = Equal?(x=w469, y="Exit") -> (x = y?=w467:bool)
      }
      event Panel Close? {
        n206 = event-data() -> ()  [unwired: 1 in, 1 out]
        n207 = Call Chain() -> (call chain=w474:string[])
        n208 = Array Size(array=w474) -> (size(s)=w473:i32)
        n209 = case shown="2, 默认" w473 {
          tunnel: w472 -> [w478 w481]
          tunnel: [w477 w480] -> w471
          tunnel: ["Panel Hidden" ("Message") "Exit Prepare" ("Message")] -> w470
          frame 2, Default {
            n210 = Unbundle By Name(w478) -> ("Message"=w477:refnum<queue>)
          }
          frame 1 {
            n211 = Unbundle By Name(w481) -> ("Message"=w480:refnum<queue>)
          }
        }
        n212 = call "Queue In.vi"("Message"=w470, "Queue In"=w471) -> ()  [unwired: 8 in, 2 out]
        n213 = event-data("Discard?"=TRUE ("放弃？")) -> ()  [unwired: 1 in, 1 out]
      }
      event "Simulation Start": Value Change {
        n214 = event-data() -> ("CtlRef"=w484:refnum<vi>)  [unwired: 1 in]
        n215 = Unbundle By Name(w486) -> ("Data"=w485:refnum<queue>)
        n216 = property class="Bool (严格)"(reference=w484) -> ("Label.Text"=w483:string)  [unwired: 1 in, 2 out]
        n217 = call "Queue In.vi"("Data"="Simulation Start", "Message"=w483, "Queue In"=w485) -> ()  [unwired: 7 in, 2 out]
      }
      event "Input": Value Change {
        n218 = event-data() -> ()  [unwired: 1 in, 6 out]
        n219 = Unbundle By Name(w489) -> ("Data"=w488:refnum<queue>)
        n220 = call "Queue In.vi"("Message"="Dispaly", "Queue In"=w488) -> ()  [unwired: 8 in, 2 out]
      }
      event "Single Simulation Start": Value Change {
        n221 = event-data() -> ("CtlRef"=w492:refnum<vi>)  [unwired: 1 in]
        n222 = Unbundle By Name(w494) -> ("Data"=w493:refnum<queue>)
        n223 = property class="Bool (严格)"(reference=w492) -> ("Label.Text"=w491:string)  [unwired: 1 in, 2 out]
        n224 = call "Queue In.vi"("Data"="Single Simulation Start", "Message"=w491, "Queue In"=w493) -> ()  [unwired: 7 in, 2 out]
      }
      event "Data Load": Value Change {
        n225 = event-data() -> ("CtlRef"=w496:refnum<vi>)  [unwired: 1 in]
        n226 = Unbundle By Name(w498) -> ("Data"=w497:refnum<queue>)
        n227 = property class="Bool"(reference=w496) -> ("Label.Text"=w495:string)  [unwired: 1 in, 2 out]
        n228 = call "Queue In.vi"("Message"=w495, "Queue In"=w497) -> ()  [unwired: 8 in, 2 out]
      }
      event "Source Edit": Value Change {
        n229 = event-data() -> ("CtlRef"=w500:refnum<vi>)  [unwired: 1 in]
        n230 = Unbundle By Name(w502) -> ("UI"=w501:refnum<queue>)
        n231 = property class="Bool"(reference=w500) -> ("Label.Text"=w499:string)  [unwired: 1 in, 2 out]
        n232 = call "Queue In.vi"("Message"=w499, "Queue In"=w501) -> ()  [unwired: 8 in, 2 out]
      }
      event "Source List": Value Change {
        n233 = event-data() -> ()  [unwired: 1 in, 1 out]
        n234 = Unbundle By Name(w505) -> ("Data"=w504:refnum<queue>)
        n235 = call "Queue In.vi"("Message"="Data Load,Dispaly", "Queue In"=w504) -> ()  [unwired: 8 in, 2 out]
      }
      event "Value", "Bool": Value Change {
        n236 = event-data() -> ("CtlRef"=w509:refnum<vi>)  [unwired: 1 in]
        n237 = property class="Ctl"(reference=w509) -> ("Label.Text"=w506:string)  [unwired: 1 in, 2 out]
        n238 = Unbundle By Name(w508) -> ("Data"=w507:refnum<queue>)
        n239 = call "Queue In.vi"("Message"=w506, "Queue In"=w507) -> ()  [unwired: 8 in, 2 out]
      }
      event "Panel Show": Value Change {
        n240 = event-data() -> ("CtlRef"=w511:refnum<vi>)  [unwired: 1 in]
        n241 = Unbundle By Name(w513) -> ("Message"=w512:refnum<queue>)
        n242 = property class="Bool"(reference=w511) -> ("Label.Text"=w510:string)  [unwired: 1 in, 2 out]
        n243 = call "Queue In.vi"("Message"=w510, "Queue In"=w512) -> ()  [unwired: 8 in, 2 out]
      }
      event "Data List": Value Change {
        n244 = event-data() -> ()  [unwired: 1 in, 1 out]
        n245 = Unbundle By Name(w516) -> ("Data"=w515:refnum<queue>)
        n246 = call "Queue In.vi"("Message"="Dispaly", "Queue In"=w515) -> ()  [unwired: 8 in, 2 out]
      }
    }
  }
  n247 = call "000 Driver Message.vi"("Queue In"=w6) -> ("error out"=w9:errorcluster)  [unwired: 8 in, 2 out]
  n248 = call "Queue Release.vi"("error in (no error)"=w12, "Queue In"=w13) -> ("error out"=w10:errorcluster)  [unwired: 9 in]
  n249 = call "Queue Release.vi"("error in (no error)"=w20, "Queue In"=w21) -> ("error out"=w17:errorcluster)  [unwired: 9 in]
  n250 = Unregister For Events(event registration refnum=w23) -> (error out=w22:errorcluster)  [unwired: 1 in]
  n251 = Destroy User Event(user event=w8, error in=w22) -> (error out=w18:errorcluster)
  n252 = Call Chain() -> (call chain=w15:string[])
  n253 = Merge Errors(w18, w17, w9, w10) -> (w16:errorcluster)
  n254 = Array Size(array=w15) -> (size(s)=w14:i32)
  n255 = case shown="2.." w14 {
    tunnel: w16 -> [_ w517]
    frame 0, Default {
    }
    frame 2.. {
      n256 = invoke class="VI" method="FP.Close"(error in=w517) -> ()  [unwired: 2 in, 3 out]
    }
  }
